vi "GetType.vi"(8 "error in (no error)":errorcluster, 11 "Configure DisSlope Msg":refnum<class "Configure DisSlope Msg.lvclass">) -> (0 "error out":errorcluster, 2 "Data Sample":variant, 3 "Configure DisSlope Msg":refnum<class "Configure DisSlope Msg.lvclass">)   [LabVIEW 2015, in "CS++MCS.lvlib" / "Configure DisSlope Msg.lvclass"]
uses:
  Configure DisSlope Msg.lvclass
  Configure DisSlope Msg.lvclass/Configure DisSlope Msg.ctl
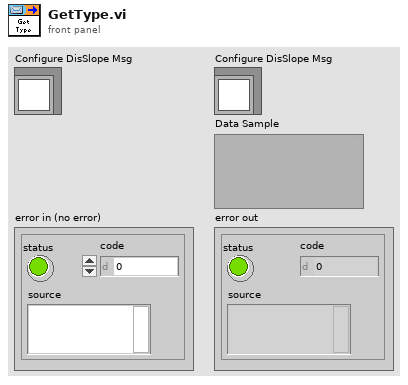
[diagram p1: front panel]
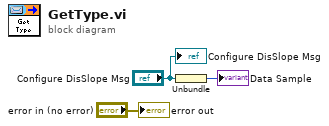
[diagram p0: block diagram]
diagram:
  n1 = Unbundle("Configure DisSlope Msg") -> (→"Data Sample":u16)
  "error out" <- "error in (no error)"
  "Configure DisSlope Msg" <- "Configure DisSlope Msg"
